vi "Write.vi"(8 "error in (no error)":errorcluster, 10 "Input":variant, 11 "DAQmx AO in":refnum<class "DAQmx AO.lvclass">) -> (0 "error out":errorcluster, 3 "DAQmx AO out":refnum<class "DAQmx AO.lvclass">)   [LabVIEW 2017, in "DAQmx AO.lvclass"]
uses:
  DAQmx AO.lvclass
  DAQmx/DAQmx.lvclass
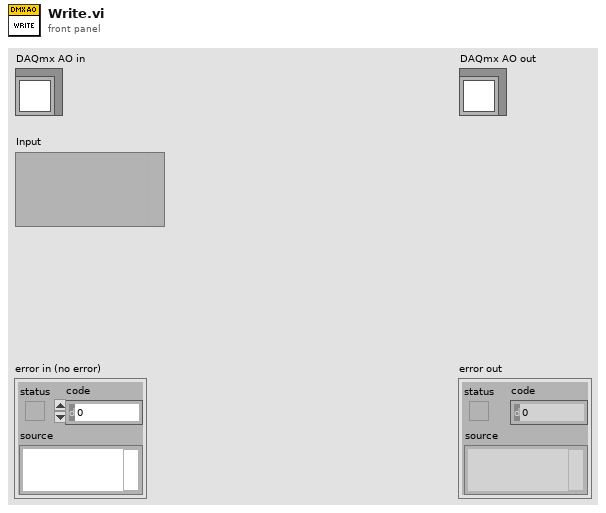
[diagram p1: front panel]
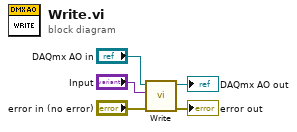
[diagram p0: block diagram]
diagram:
  n1 = call-parent "Write.vi"("error in (no error)"="error in (no error)", "Input"="Input", "DAQmx in"="DAQmx AO in") -> ("error out"=→"error out":errorcluster, "DAQmx out"=→"DAQmx AO out":refnum<class "DAQmx AO.lvclass">)  [unwired: 7 in]
